vi "Read Thermocouple Type.vi"(8 "error in":errorcluster, 11 "thermocouple channel in":refnum<class "Thermocouple Channel.lvclass">) -> (0 "error out":errorcluster, 2 "thermocouple type":T1, 3 "thermocouple channel out":refnum<class "Thermocouple Channel.lvclass">)   [LabVIEW 2020, in "Scan Engine Scripting.lvlib" / "Thermocouple Channel.lvclass"]
uses:
  Thermocouple Channel.lvclass
  Thermocouple Type.ctl
  Thermocouple Channel.lvclass/Thermocouple Channel.ctl
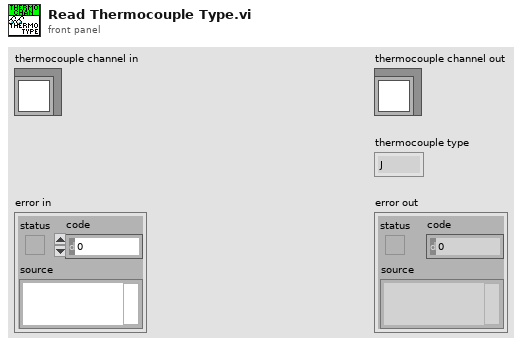
[diagram p1: front panel]
types:
  T1 = typedef "Scan Engine Scripting.lvlib/Thermocouple Channel.lvclass/Thermocouple Type.ctl" = enum16{"J", "K", "T", "E", "R", "S", "N", "B"}
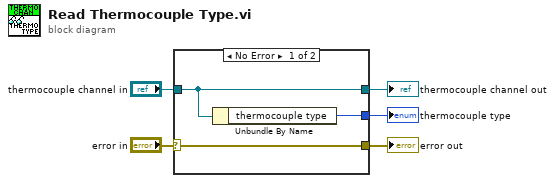
[diagram p0: block diagram]
diagram:
  n1 = case shown="No Error" "error in" {
    selector: "error in" -> [w8 w9]
    tunnel: [w8 w9] -> w4
    tunnel: [w7 w10] -> w2
    tunnel: "thermocouple channel in" -> [w7 w10]
    tunnel: [w6 _] -> w1
    frame No Error {
      n2 = Unbundle By Name(w7) -> ("thermocouple type"=w6:T1)
    }
    frame Error {
    }
  }
  "error out" <- w4
  "thermocouple channel out" <- w2
  "thermocouple type" <- w1
